vi "Write Network Slave.vi"(8 "error in (no error)":errorcluster, 10 "Network Slave":refnum<class "Network Slave.lvclass">, 11 "Modbus Slave in":refnum<class "Modbus Slave.lvclass">) -> (0 "error out":errorcluster, 3 "Modbus Slave out":refnum<class "Modbus Slave.lvclass">)   [LabVIEW 2021, in "Modbus Slave.lvclass"]
uses:
  Modbus Slave.lvclass
  Modbus Slave.lvclass/Modbus Slave.ctl
  Network Protocol/Network Slave/Network Slave.lvclass
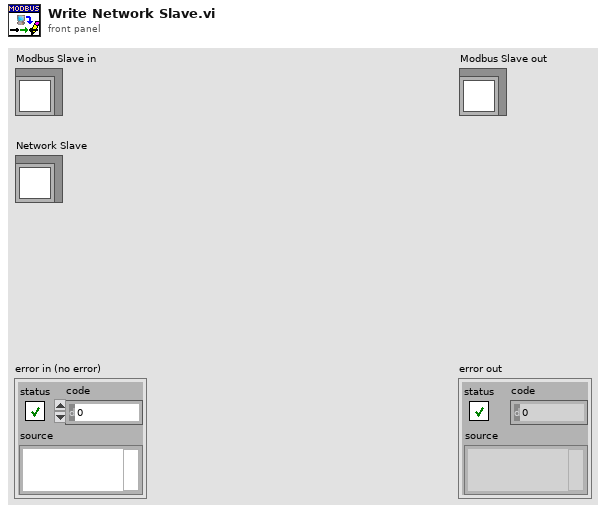
[diagram p1: front panel]
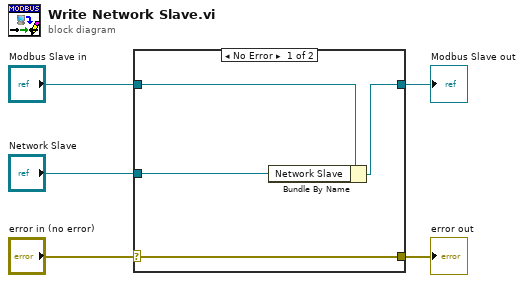
[diagram p0: block diagram]
diagram:
  n1 = case shown="No Error" "error in (no error)" {
    selector: "error in (no error)" -> [w9 w10]
    tunnel: [w9 w10] -> w4
    tunnel: [w7 w11] -> w2
    tunnel: "Modbus Slave in" -> [w8 w11]
    tunnel: "Network Slave" -> [w6 _]
    frame No Error {
      n2 = Bundle By Name(cluster=w8, "Network Slave"=w6) -> (w7:refnum<class "Modbus Slave.lvclass">)
    }
    frame Error {
    }
  }
  "error out" <- w4
  "Modbus Slave out" <- w2
